vi "pH edit buffer list.vi"(3 "index":i32) -> (1 "Buffers out":T1(array[cluster]) {"V/T" format="%.2f"; "Buffer" format="%.2f"})   [LabVIEW 2012]
uses:
  global scale array.vi
panel:
  in  "Cancel Button":bool
  in  "OK Button":bool
  in  "Buffers":T1(array[cluster]) {"V/T" format="%.2f"; "Buffer" format="%.2f"}
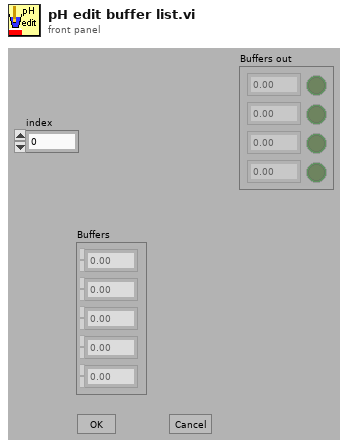
[diagram p1: front panel]
types:
  T1 = cluster{"Buffer":dbl, "Calibrated":bool, "V/T":dbl}[]
  T2 = typedef "calib array.ctl" = T3[]
  T3 = typedef "conversion.ctl" = cluster{"conversion matrix":sgl[][], "units":string, "name":string, "scale type":T4, "offset (volts)":dbl, "second channel":i8, "correspondence table":T5, "offset (physical units)":dbl, "pH scale":T6, "D.O.":T7}
  T4 = typedef "scale type.ctl" = enum16{"Volts", "Polynomial", "Correspondence Table", "pH", "Dissolved Oxygen", "Quadratic"}
  T5 = typedef "correspondence table.ctl" = cluster{"physical units":dbl, "volts":dbl}[]
  T6 = typedef "pH scale.ctl" = cluster{"Buffers":cluster{"Buffer":dbl, "Calibrated":bool, "V/T":dbl}[], "Temperature":dbl}
  T7 = typedef "DO scale.ctl" = cluster{"Temperature":dbl, "K":dbl, "barometric pressure":dbl}
  T8 = cluster{"Buffer":dbl, "Calibrated":bool, "V/T":dbl}
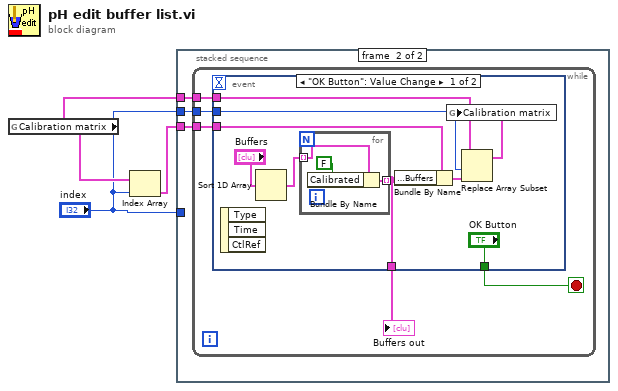
[diagram p0: block diagram]
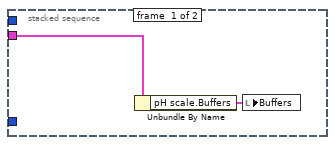
[diagram p2: hidden frame]
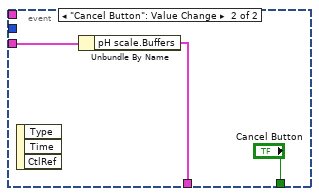
[diagram p3: hidden frame]
diagram:
  n1 = global read "global scale array.vi" "Calibration matrix"() -> (w3:T2)
  n2 = Index Array(array=w3, index="index") -> (element=w2:T3)
  n3 = stacked-sequence {
    tunnel: "index" -> [_ _]
    tunnel: w2 -> [w4 w8]
    tunnel: w3 -> [_ w7]
    tunnel: "index" -> [_ w6]
    frame #0 {
      n4 = Unbundle By Name(w4) -> ("pH scale.Buffers"=w5:T1)
      n5 = local write "Buffers"(w5) -> ()
    }
    frame #1 {
      n6 = while {
        tunnel: w8 -> [w13]
        tunnel: w7 -> [w12]
        tunnel: w6 -> [w11]
        stop <- w10 stop-if-true
        n7 = event shown="[0] \"OK Button\": Value Change" {
          selector: _ -> [_ _]
          dyn-events: _ -> [_ _]
          timeout: _ -> [_ _]
          tunnel: w13 -> [w22 w27]
          tunnel: w12 -> [w21 _]
          tunnel: w11 -> [w20 _]
          tunnel: ["OK Button" "Cancel Button"] -> w10
          tunnel: [w16 w26] -> w9
          event "OK Button": Value Change {
            n8 = event-data() -> ()  [unwired: 1 in, 3 out]
            n9 = Sort 1D Array(array="Buffers") -> (sorted array=w14:T1)
            n10 = for {
              tunnel: w14 -> [w25] mode=indexing
              tunnel: [w23] -> w16 mode=indexing
              n11 = Bundle By Name(cluster=w25, "Calibrated"=FALSE) -> (w23:T8)
            }
            n12 = Bundle By Name(cluster=w22, "pH scale.Buffers"=w16) -> (w17:T3)
            n13 = Replace Array Subset(array=w21, new element=w17, index=w20) -> (w19:T2)
            n14 = global write "global scale array.vi" "Calibration matrix"(w19) -> ()
          }
          event "Cancel Button": Value Change {
            n15 = event-data() -> ()  [unwired: 1 in, 3 out]
            n16 = Unbundle By Name(w27) -> ("pH scale.Buffers"=w26:T1)
          }
        }
        "Buffers out" <- w9
      }
    }
  }
